vi "OracleBusyDialog.vi"() -> ()   [LabVIEW 2017, in "Server.lvlib" / "Oracle.lvlib"]
doc: "This Dialog indicates, that Oracle is still running a Query that can't be aborted. It shows the user that this is expected and the application did not randomly crash. He can avoid the waiting by killing the application in Task Manager. This Dialog is opened when the application stops, and aborted (via VI server) when the Oracle Loop has finished its execution. If this VI is not aborted within 60 seconds, it will return a Timeout error telling that there seems to be a critical hang in the Oracle Loop and User should kill the application in Task Manager."
uses:
  Oracle.lvlib
  <vilib>/Utility/error.llb/Error Cluster From Error Code.vi
  <vilib>/ErrorRing/Error Ring.xnode
panel:
  out "Horizontal Progress Bar":i32(slide) scale=0.0..1000.0
  # "WAITING FOR ORACLE TO FINISH..."
  # "This may take up to 60 seconds!"
  # "Please be patient or kill application in Task Manager."
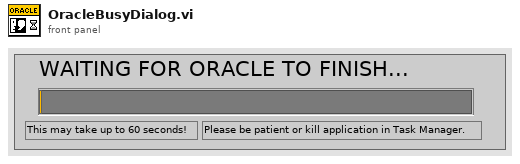
[diagram p1: front panel]
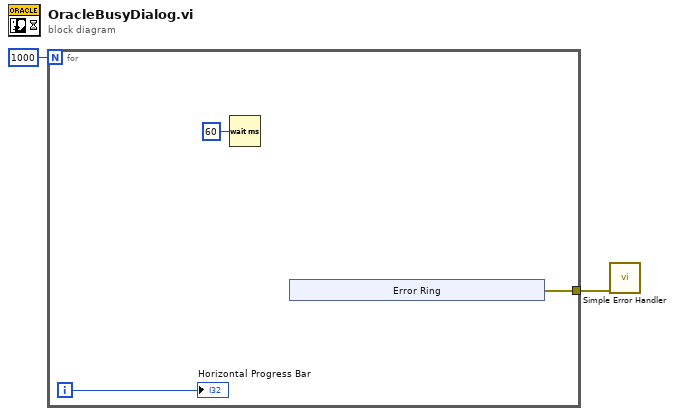
[diagram p0: block diagram]
diagram:
  n1 = for {
    N: 1000 -> [_]
    tunnel: [w3] -> w1
    i -> [w4]
    n2 = Wait (ms)(milliseconds to wait=u32 60) -> ()  [unwired: 1 out]
    n3 = xnode "Error Ring"() -> ("error out"=w3:errorcluster)
    "Horizontal Progress Bar" <- w4
  }
  n4 = call <vilib>:"Simple Error Handler.vi"("error in (no error)"=w1) -> ()  [unwired: 4 in, 5 out]
